vi "Cancel.vi"(8 "error in (no error)":errorcluster, 11 "Future in":refnum<class "Future.lvclass">) -> (0 "error out":errorcluster)   [LabVIEW 2017, in "Futures.lvlib" / "Future.lvclass"]
doc: "Cancel the future rendering it invalid.\n\nThis cleans up the resources for active futures and gives task handlers the chance to cancel prematurely."
uses:
  Future.lvclass
  Future.lvclass/Future.ctl
  Task/Task.lvclass
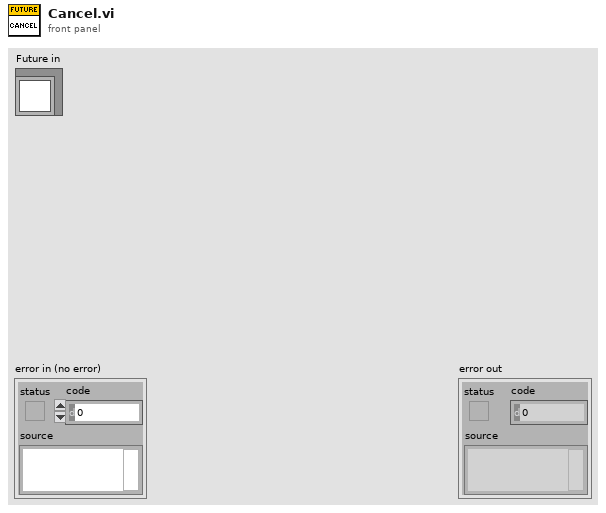
[diagram p1: front panel]
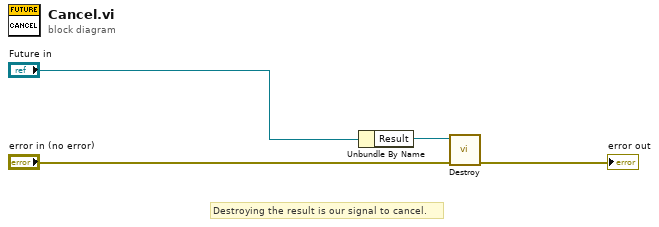
[diagram p0: block diagram]
diagram:
  # "Destroying the result is our signal to cancel."
  n1 = Unbundle By Name("Future in") -> ("Result"=w1:refnum<class "Task.lvclass">)
  n2 = call "Destroy.vi"("error in (no error)"="error in (no error)", "Result in"=w1) -> ("error out"=→"error out":errorcluster)  [unwired: 9 in]
